vi "Billede_til_string_og_tilbage.vi"() -> ()   [LabVIEW 2018]
uses:
  <vilib>/vision/NI_Vision_Development_Module.lvlib
panel:
  in  "File Path":path=path "U:/"
  out "array":u8[][](array[numeric])
  out "Image Pixels (U8)":u8[][](array[numeric])
  out "Intensity Graph 5":u16[][](graph)
  out "Intensity Graph 4":u8[][](graph)
  in  "Rotation \nOrientation":bool
  out "Intensity Graph 3":u8[][](graph)
  in  "stop":bool
  out "Original":T1(plugin-control)
  out "Luminance Plane":T1(plugin-control)
  out "Red Plane (as grayscale)":T1(plugin-control)
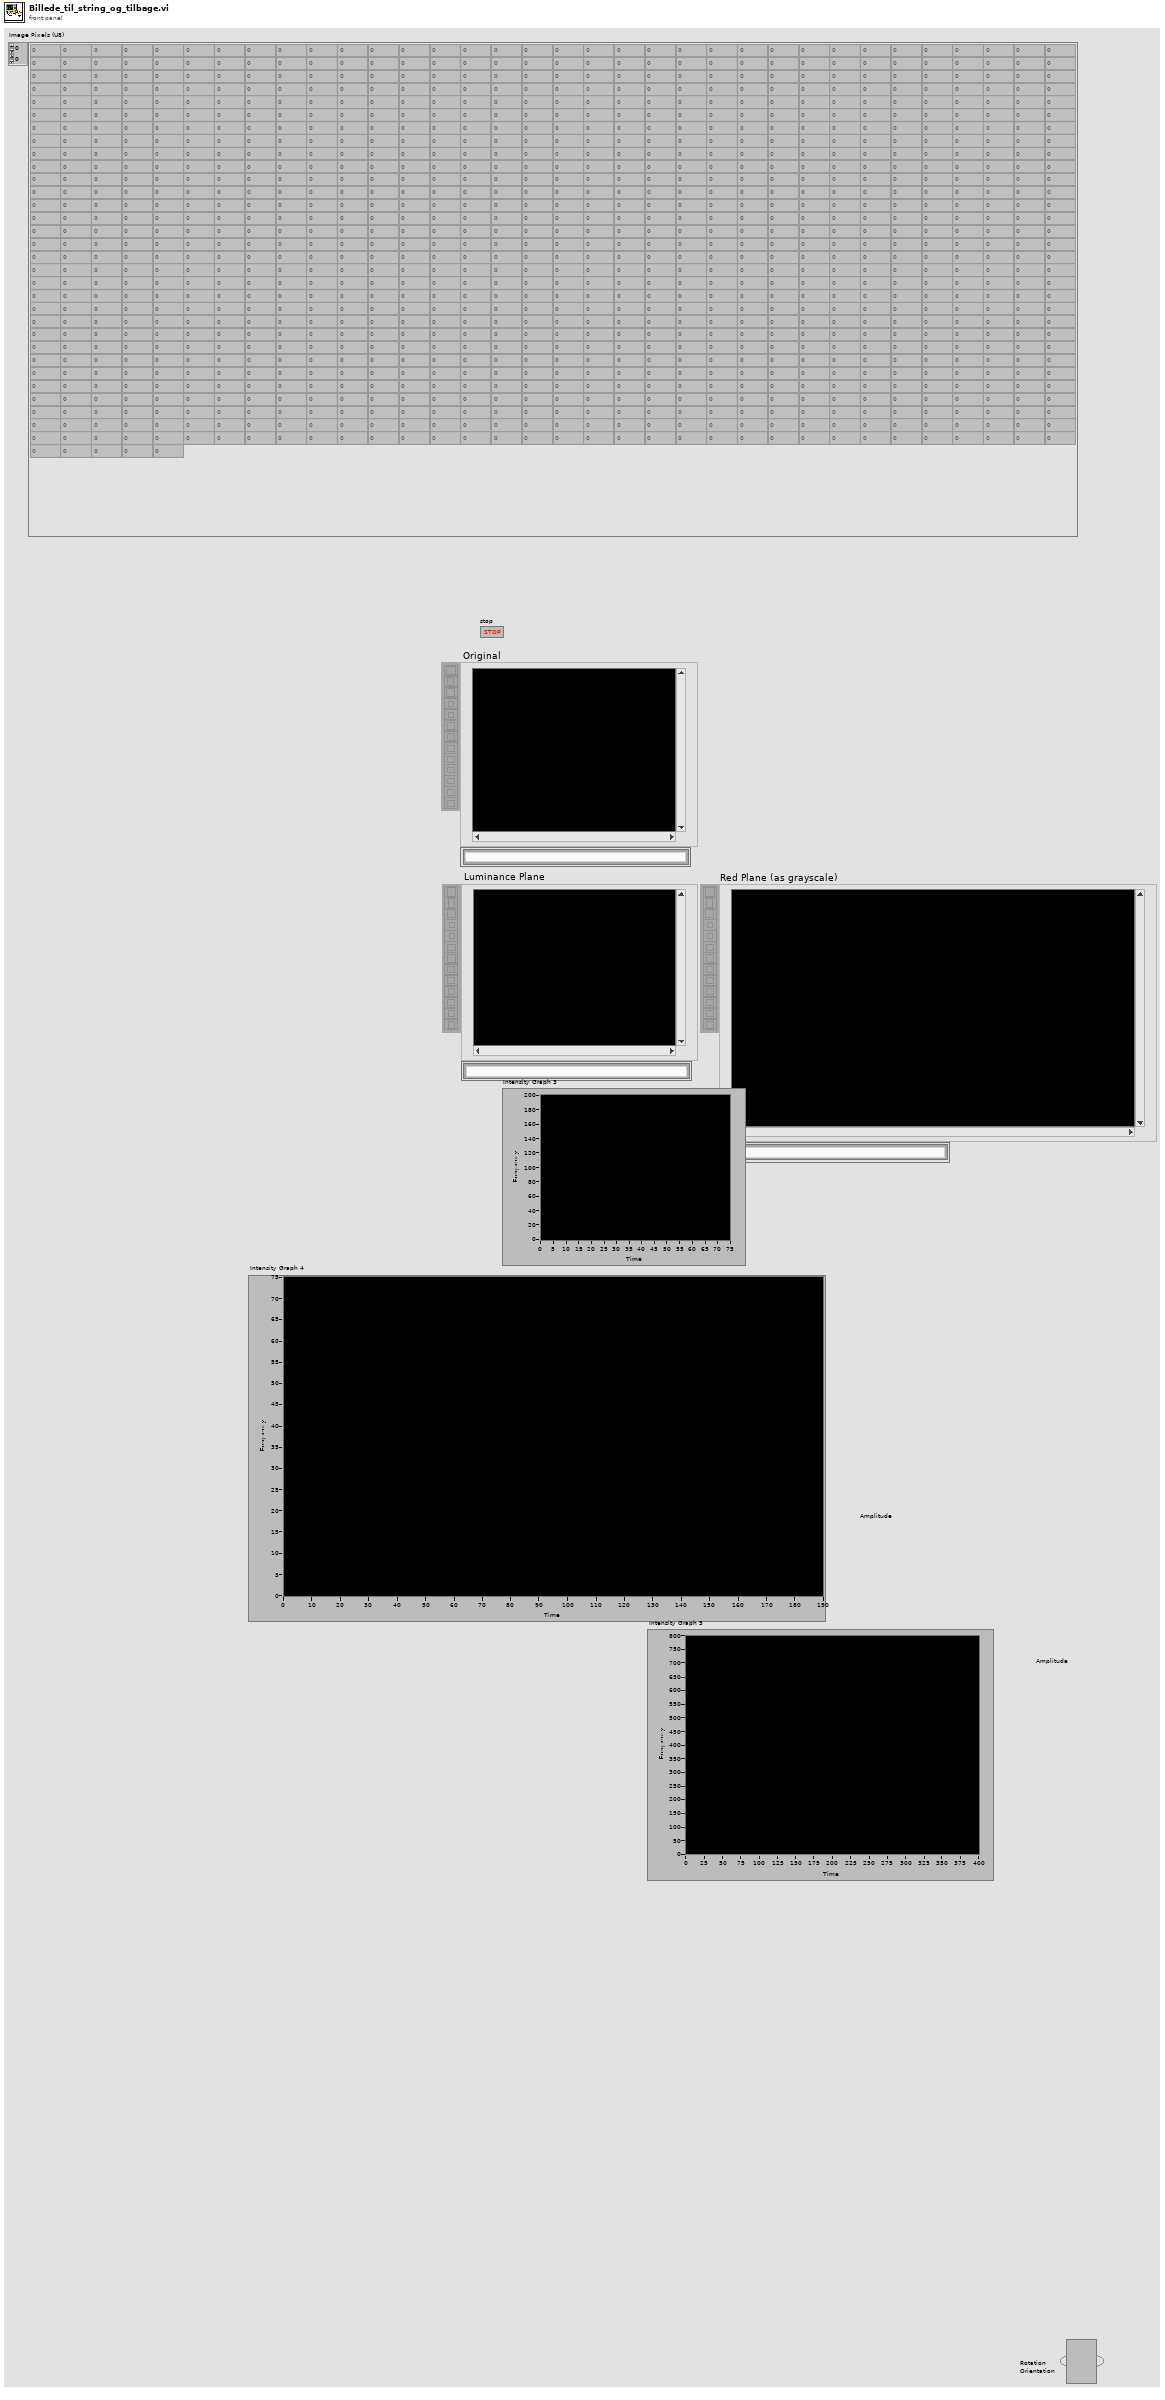
[diagram p1: front panel]
types:
  T1 = typedef "IMAQ Image.ctl" = refnum<image>
  T2 = typedef "Image Type" = u32
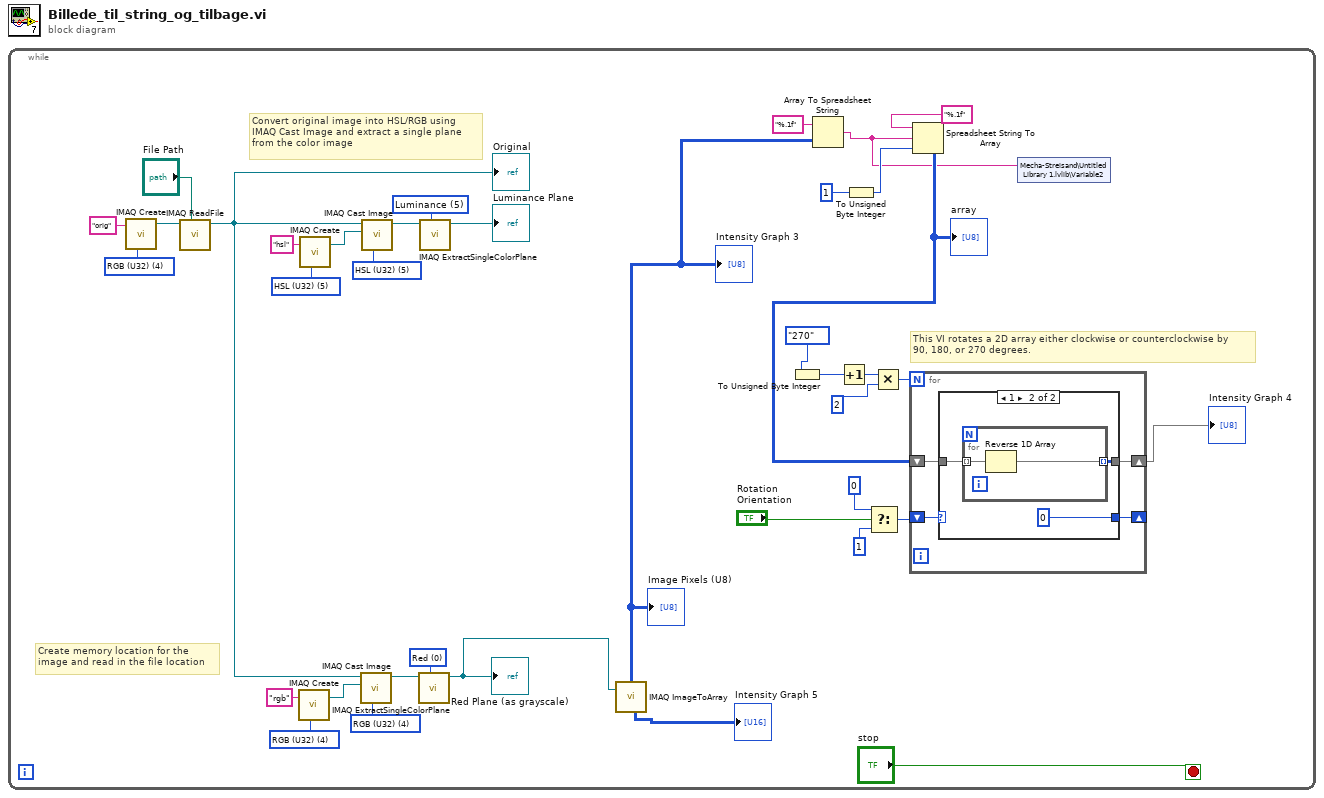
[diagram p0: block diagram]
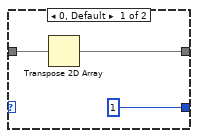
[diagram p2: hidden frame]
diagram:
  n1 = while {
    stop <- "stop" stop-if-true
    w22 = T2 4 items=["Grayscale (U8)", "Grayscale (I16)", "Grayscale (SGL)", "Complex (CSG)", "RGB (U32)", "HSL (U32)", "RGB (U64)"] ("Image Type")
    w30 = 0 items=["Red", "Green", "Blue", "Hue", "Saturation", "Luminance", "Value", "Intensity"] ("Color Plane")
    w28 = T2 4 items=["Grayscale (U8)", "Grayscale (I16)", "Grayscale (SGL)", "Complex (CSG)", "RGB (U32)", "HSL (U32)", "RGB (U64)"] ("Image Type")
    w27 = T2 4 items=["Grayscale (U8)", "Grayscale (I16)", "Grayscale (SGL)", "Complex (CSG)", "RGB (U32)", "HSL (U32)", "RGB (U64)"] ("Image Type")
    w32 = 5 items=["Red", "Green", "Blue", "Hue", "Saturation", "Luminance", "Value", "Intensity"] ("Color Plane")
    w34 = T2 5 items=["Grayscale (U8)", "Grayscale (I16)", "Grayscale (SGL)", "Complex (CSG)", "RGB (U32)", "HSL (U32)", "RGB (U64)"] ("Image Type")
    w35 = T2 5 items=["Grayscale (U8)", "Grayscale (I16)", "Grayscale (SGL)", "Complex (CSG)", "RGB (U32)", "HSL (U32)", "RGB (U64)"] ("Image Type")
    # "This VI rotates a 2D array either clockwise or counterclockwise by\n90, 180, or 270 degrees."
    # "Convert original image into HSL/RGB using\nIMAQ Cast Image and extract a single plane\nfrom the color image"
    # "Create memory location for the \nimage and read in the file location"
    n2 = call "IMAQ Create"("Image Name"="orig", "Image Type"=w22) -> ("New Image"=w24:T1)  [unwired: 2 in, 2 out]
    n3 = call "IMAQ ReadFile"("File Path"="File Path", "Image"=w24) -> ("Image Out"=w21:T1)  [unwired: 3 in, 6 out]
    "Original" <- w21
    n4 = call "IMAQ Create"("Image Name"="rgb", "Image Type"=w27) -> ("New Image"=w25:T1)  [unwired: 2 in, 2 out]
    n5 = call "IMAQ Create"("Image Name"="hsl", "Image Type"=w35) -> ("New Image"=w37:T1)  [unwired: 2 in, 2 out]
    n6 = call "IMAQ Cast Image"("Image Type"=w28, "Image Dst"=w25, "Image Src"=w21) -> ("Image Dst Out"=w29:T1)  [unwired: 3 in, 5 out]
    n7 = call "IMAQ Cast Image"("Image Type"=w34, "Image Dst"=w37, "Image Src"=w21) -> ("Image Dst Out"=w33:T1)  [unwired: 3 in, 5 out]
    n8 = call "IMAQ ExtractSingleColorPlane"("Color Plane"=w30, "Image Src"=w29) -> ("Image Dst Out"=w19:T1)  [unwired: 2 in, 7 out]
    "Red Plane (as grayscale)" <- w19
    n9 = call "IMAQ ExtractSingleColorPlane"("Color Plane"=w32, "Image Src"=w33) -> ("Image Dst Out"=→"Luminance Plane":T1)  [unwired: 2 in, 7 out]
    n10 = call "IMAQ ImageToArray"("Image"=w19) -> ("Image Pixels (U16)"=→"Intensity Graph 5":u16[][], "Image Pixels (U8)"=w17:u8[][])  [unwired: 3 in, 3 out]
    "Intensity Graph 3" <- w17
    "Image Pixels (U8)" <- w17
    n11 = To Unsigned Byte Integer(number=enum8{"90", "180", "270"}."270" ("Rotation")) -> (unsigned 8bit integer=w5:u8)
    n12 = Array To Spreadsheet String(array=w17, 3:"%.1f" ("format string")) -> (spreadsheet string=w1:string)  [unwired: 1 in]
    n13 = Increment(x=w5) -> (x+1=w7:u8)
    n14 = To Unsigned Byte Integer(number=u8 1) -> (unsigned 8bit integer=w16:u8)
    n15 = Select(t=u8 0, s="Rotation \nOrientation", f=u8 1) -> (s? t:f=w9:u8)
    n16 = Multiply(x=w7, y=u8 2) -> (x*y=w8:u8)
    n17 = Spreadsheet String To Array(format string="%.1f", spreadsheet string=w1, array type (2D Dbl)=w16) -> (array=w2:u8[][])  [unwired: 1 in]
    "array" <- w2
    n18 = for {
      N: w8 -> [_]
      shift-right: [w41] -> w4
      shift-left: w2 -> [w42]
      shift-right: [w39] -> _
      shift-left: w9 -> [w40]
      n19 = case shown="1" w40 {
        tunnel: w42 -> [w44 w48]
        tunnel: [w45 w47] -> w41
        tunnel: [u8 1 u8 0] -> w39
        frame 0, Default {
          n20 = Transpose 2D Array(2D array=w44) -> (transposed array=w45:u8[][])
        }
        frame 1 {
          n21 = for {
            tunnel: w48 -> [w50] mode=indexing
            tunnel: [w49] -> w47 mode=indexing
            n22 = Reverse 1D Array(array=w50) -> (reversed array=w49:u8[])
          }
        }
      }
    }
    "Intensity Graph 4" <- w4
    n23 = shared-variable "Mecha-Streisand\\Untitled Library 1.lvlib\\Variable2"(w1) -> ()  [unwired: 1 in, 1 out]
  }
